vi "Stop Core.vi"(10 "final error code":i32, 11 "Filled Text Fields Actor in":refnum<class "Filled Text Fields Actor.lvclass">) -> (3 "Filled Text Fields Actor out":refnum<class "Filled Text Fields Actor.lvclass">)   [LabVIEW 2017, in "Filled Text Fields Actor.lvlib" / "Filled Text Fields Actor.lvclass"]
doc: "(<B>Filename</B>: Actor Framework.lvlib:Actor.lvclass:Stop Core.vi)\n\nDefines what the actor does before it stops. Use the <B>final error code</B> input to determine whether the actor shut down in response to an error.\n\nBy default, this method does nothing. A descendant class may override it to define behavior, such as shutting down any processes the actor initiated in its override of the Actor Core method."
uses:
  Filled Text Fields Actor.lvclass
  <vilib>/event_ctls.llb/usereventprio.ctl
  Filled Text Fields Actor.lvclass/Filled Text Fields Actor.ctl
  <vilib>/ActorFramework/Actor/Actor.lvclass
  Theme/Theme/Theme.lvclass
  Data/Data.lvclass
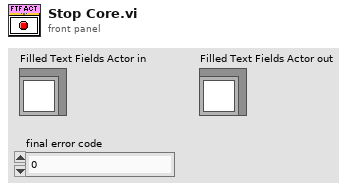
[diagram p1: front panel]
types:
  T1 = typedef "usereventprio.ctl" = enum32{"high priority", "normal priority"}
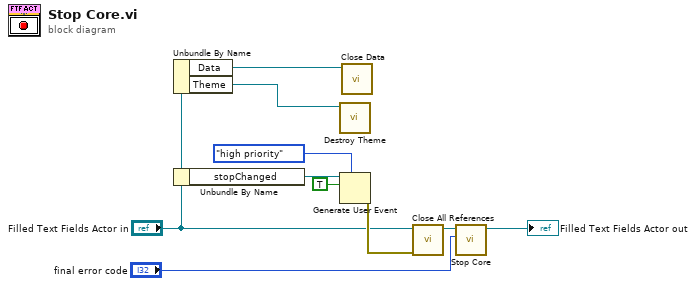
[diagram p0: block diagram]
diagram:
  n1 = Unbundle By Name("Filled Text Fields Actor in") -> ("Data"=w1:refnum<class "Data.lvclass">, "Theme"=w2:refnum<class "Theme.lvclass">)
  n2 = Unbundle By Name("Filled Text Fields Actor in") -> ("stopChanged"=w8:refnum<user-event>)
  n3 = call "Destroy Theme.vi"("Theme in"=w2) -> ()  [unwired: 10 in, 1 out]
  n4 = Generate User Event(priority (normal)=usereventprio."high priority", user event=w8, event data cluster=TRUE ("event data")) -> (error out=w4:errorcluster)  [unwired: 1 in, 1 out]
  n5 = call "Close Data.vi"("Data in"=w1) -> ()  [unwired: 10 in, 1 out]
  n6 = call "Close All References.vi"("error in (no error)"=w4, "Filled Text Fields Actor in"="Filled Text Fields Actor in") -> ("Filled Text Fields Actor out"=w5:refnum<class "Filled Text Fields Actor.lvclass">)  [unwired: 8 in, 1 out]
  n7 = call-parent "Stop Core.vi"("final error code"="final error code", "Actor in"=w5) -> ("Actor out"=→"Filled Text Fields Actor out":refnum<class "Filled Text Fields Actor.lvclass">)  [unwired: 9 in]
